vi "pack Galvo data-test.vi"() -> ()   [LabVIEW 2015]
uses:
  DRAM data index.ctl
panel:
  out "Packed data":i32
  out "output valid?":bool
  in  "stop":bool
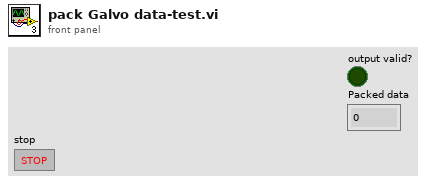
[diagram p1: front panel]
types:
  T1 = typedef "DRAM data index.ctl" = enum16{"Numeric 1", "Numeric 2", "Numeric 3", "Numeric 4", "Numeric 5", "Numeric 6", "Numeric 7", "Numeric 8", "Numeric 9", "Numeric 10", "Numeric 11", "Numeric 12", "Numeric 13", "Numeric 14", "Numeric 15", "Numeric 16"}
  T2 = cluster{"Numeric 1":u32, "Numeric 2":u32, "Numeric 3":u32, "Numeric 4":u32, "Numeric 5":u32, "Numeric 6":u32, "Numeric 7":u32, "Numeric 8":u32, "Numeric 9":u32, "Numeric 10":u32, "Numeric 11":u32, "Numeric 12":u32, "Numeric 13":u32, "Numeric 14":u32, "Numeric 15":u32, "Numeric 16":u32}
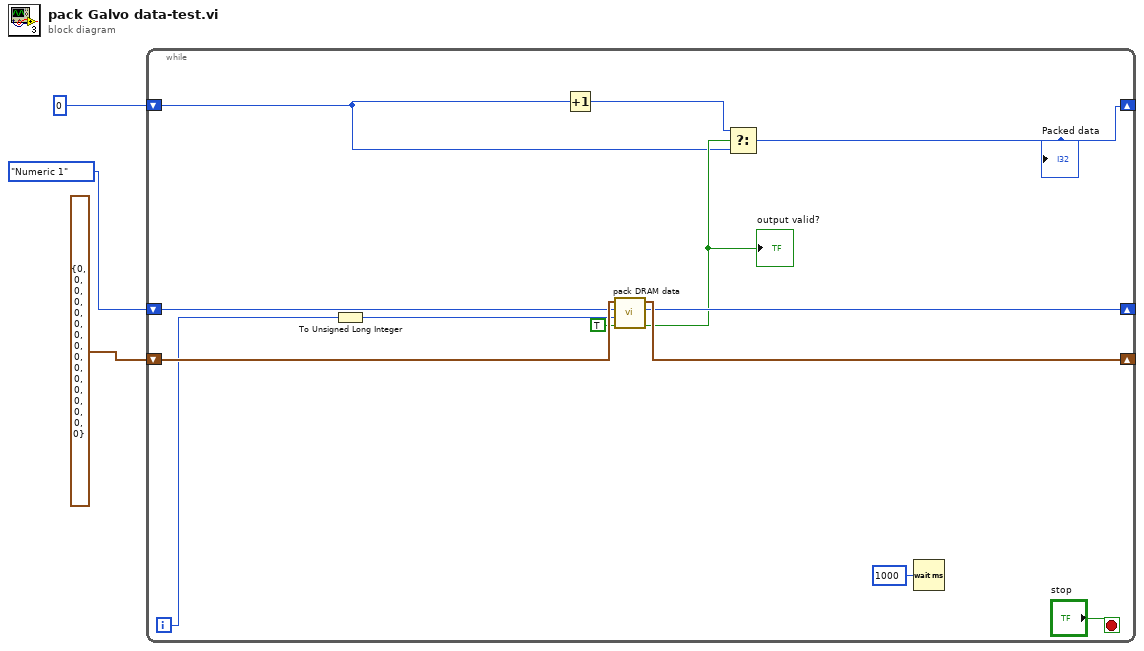
[diagram p0: block diagram]
diagram:
  n1 = while {
    shift-right: [w9] -> _
    shift-left: T2 {"Numeric 1"=0, "Numeric 2"=0, "Numeric 3"=0, "Numeric 4"=0, "Numeric 5"=0, "Numeric 6"=0, "Numeric 7"=0, "Numeric 8"=0, "Numeric 9"=0, "Numeric 10"=0, "Numeric 11"=0, "Numeric 12"=0, "Numeric 13"=0, "Numeric 14"=0, "Numeric 15"=0, "Numeric 16"=0} ("packer in") -> [w14]
    shift-right: [w8] -> _
    shift-left: DRAM_data_index."Numeric 1" ("Galvo index in") -> [w13]
    shift-right: [w5] -> _
    shift-left: 0 -> [w6]
    i -> [w12]
    stop <- "stop" stop-if-true
    n2 = To Unsigned Long Integer(number=w12) -> (unsigned 32bit integer=w11:u32)
    n3 = Increment(x=w6) -> (x+1=w4:i32)
    n4 = call "pack DRAM data.vi"("input valid?"=TRUE, "data to be packed"=w11, "DRAM Index in"=w13, "packer in"=w14) -> ("output valid?"=w7:bool, "DRAM Index out"=w8:T1, "packer out"=w9:T2)  [unwired: 5 in]
    "output valid?" <- w7
    n5 = Select(t=w4, s=w7, f=w6) -> (s? t:f=w5:i32)
    "Packed data" <- w5
    n6 = Wait (ms)(milliseconds to wait=u32 1000) -> ()  [unwired: 1 out]
  }
